vi "Find Survey Scan Start Point.vi"(7 "Error In":errorcluster, 8 "Polygon Diameter (km)":dbl, 9 "Bearing":dbl, 10 "Points of Polygon":T1[](array[typedef]) {"Latitude" format="%#_10g"; "Longitude" format="%#_10g"}) -> (0 "Error Out":errorcluster, 1 "Start Point Lat":dbl, 2 "Start Point Lon":dbl, 3 "Start Point":T1 {"Latitude" format="%#_10g"; "Longitude" format="%#_10g"})   [LabVIEW 2014]
uses:
  Lat Long Conversion/Controls/PointLatLon.ctl
  Lat Long Conversion/Decrement Bearing.vi
  <vilib>/Analysis/NI_AAL_Geometry.lvlib
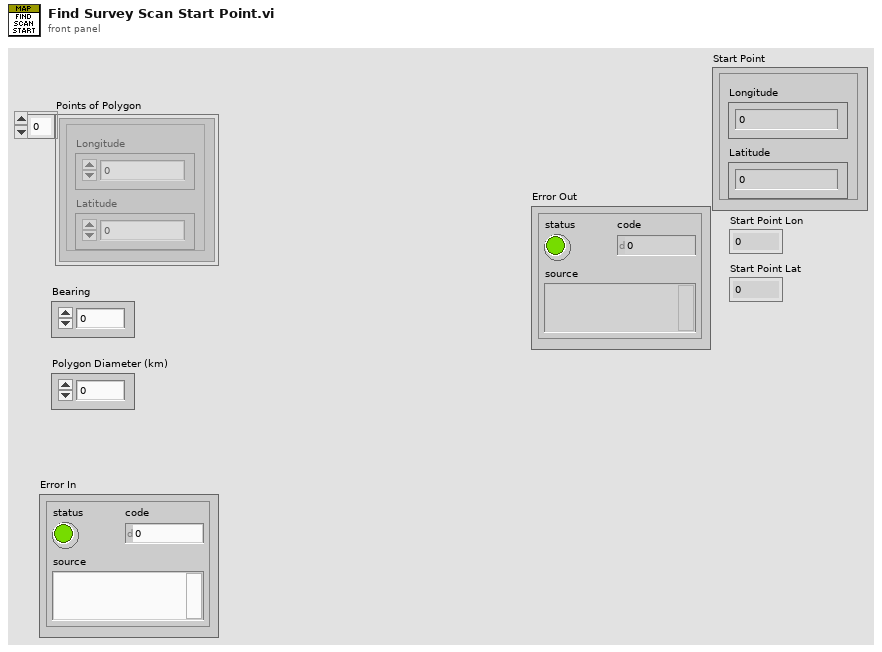
[diagram p1: front panel]
types:
  T1 = typedef "PointLatLon.ctl" = cluster{"Longitude":dbl, "Latitude":dbl}
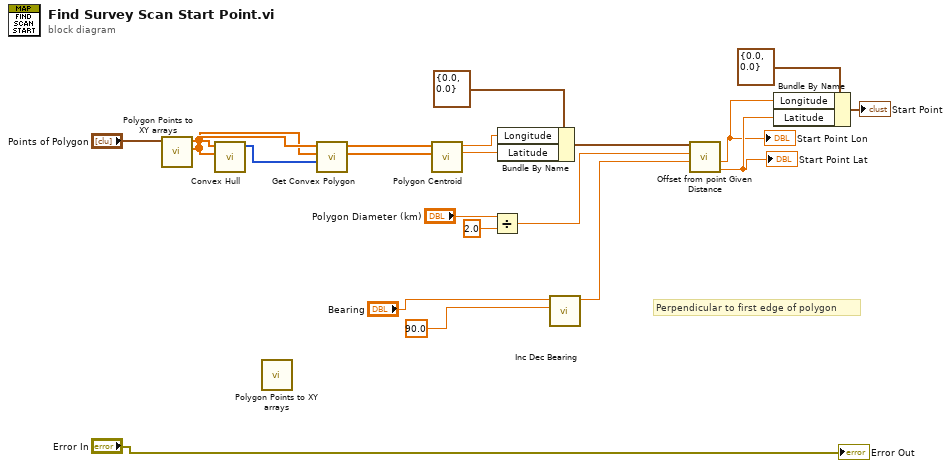
[diagram p0: block diagram]
diagram:
  # "Perpendicular to first edge of polygon"
  n1 = call "Polygon Points to XY arrays.vi"("Polygon Points"="Points of Polygon") -> ("Y Array"=w5:dbl[], "X Array"=w6:dbl[])  [unwired: 9 in]
  n2 = call <vilib>:"Convex Hull.vi"("Y"=w5, "X"=w6) -> ("Convex Hull"=w4:i32[])  [unwired: 8 in, 1 out]
  n3 = call "Polygon Points to XY arrays.vi"() -> ()  [unwired: 10 in, 2 out]
  n4 = call "Get Convex Polygon.vi"("Convex Hull Points"=w4, "y"=w5, "X"=w6) -> ("Y"=w1:dbl[], "X"=w2:dbl[])  [unwired: 7 in]
  n5 = call <vilib>:"Polygon Centroid.vi"("Y"=w1, "X"=w2) -> ("Centroid Y"=w19:dbl, "Centroid X"=w20:dbl)  [unwired: 7 in, 1 out]
  n6 = Divide(x="Polygon Diameter (km)", y=2.0) -> (x/y=w15:dbl)
  n7 = Bundle By Name(cluster=T1 {"Longitude"=0.0, "Latitude"=0.0} ("Origin Point"), "Longitude"=w20, "Latitude"=w19) -> (w18:T1)
  n8 = call-poly "Inc Dec Bearing.vi"("Decrement Value"=90.0 ("y"), "Bearing"="Bearing") -> ("New Bearing"=w8:dbl)  [unwired: 8 in, 1 out]
  n9 = call "Offset from point Given Distance.vi"("Bearing (clockwise from North)"=w8, "Distance (km)"=w15, "Origin Point"=w18) -> ("Lat of new point"=w11:dbl, "Lon of new point"=w10:dbl)  [unwired: 5 in, 2 out]
  "Start Point Lon" <- w10
  "Start Point Lat" <- w11
  n10 = Bundle By Name(cluster=T1 {"Longitude"=0.0, "Latitude"=0.0} ("Origin Point"), "Longitude"=w10, "Latitude"=w11) -> (→"Start Point":T1)
  "Error Out" <- "Error In"
